vi "Observe Data.vi"(6 "Time Stamp":timestamp, 8 "error in (no error)":errorcluster, 9 "Value":variant, 10 "Datum Name":string, 11 "Stop Process View Definition in":refnum<class "Stop Process View Definition.lvclass">) -> (0 "error out":errorcluster, 3 "Stop Process View Definition out":refnum<class "Stop Process View Definition.lvclass">)   [LabVIEW 2019, in "Stop Process View Definition.lvclass"]
doc: "<License>\nCopyright © 2017 Composed Systems, LLC | All rights reserved\nwww.composed.io\n\nAuthor: Ethan Stern <ethan.stern@composed.io>\n\nThis software is provided \"AS IS\" WITHOUT WARRANTIES, either express or implied, AND IS FOR EDUCATIONAL PURPOSES ONLY.\n</License>"
uses:
  <vilib>/gpm_packages/@cs/Car-wash/Source/Stop Process View Definition/Stop Process View Definition.lvclass
  <vilib>/gpm_packages/@cs/Car-wash/Source/Stop Process View Definition/Stop Process View Definition.lvclass/Stop Process View Definition.ctl
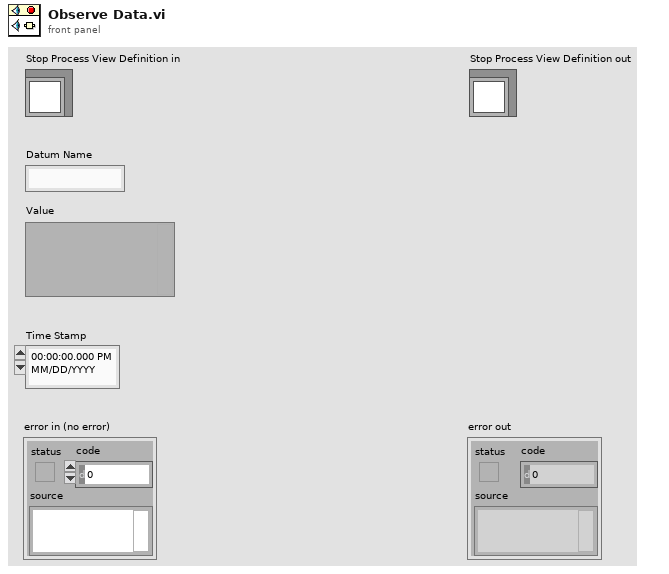
[diagram p1: front panel]
types:
  T1 = enum8{"Enabled", "Disabled", "Disabled and Grayed Out"}
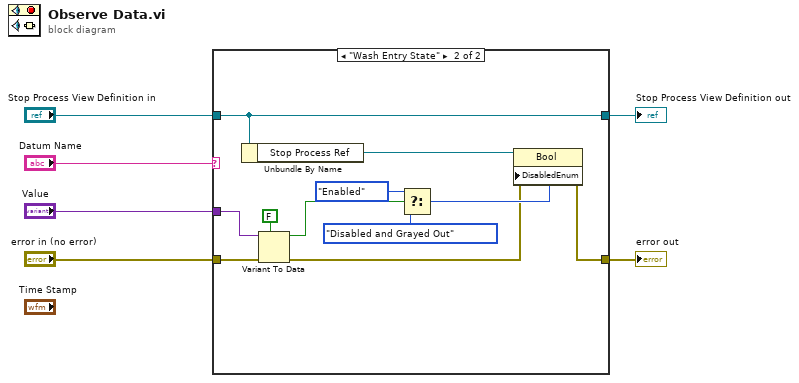
[diagram p0: block diagram]
diagram:
  n1 = case shown="\"Wash Entry State\"" "Datum Name" {
    tunnel: [w8 w16] -> w5
    tunnel: "Stop Process View Definition in" -> [w8 w16]
    tunnel: [w7 w9] -> w3
    tunnel: "error in (no error)" -> [w7 w19]
    tunnel: "Value" -> [_ w18]
    frame Default {
    }
    frame "Wash Entry State" {
      n2 = Unbundle By Name(w16) -> ("Stop Process Ref"=w15:refnum<vi>)
      n3 = Variant To Data(error in=w19, type=FALSE, Variant=w18) -> (data=w14:bool, error out=w10:errorcluster)
      n4 = Select(t=T1."Enabled", s=w14, f=T1."Disabled and Grayed Out" ("Disabled")) -> (s? t:f=w12:T1)
      n5 = property class="Bool"(reference=w15, error in=w10, "DisabledEnum"=w12) -> (error out=w9:errorcluster)  [unwired: 1 out]
    }
  }
  "error out" <- w3
  "Stop Process View Definition out" <- w5
